vi "Sensors_GCFS.vi"(0 "?":T2={"Core"={"Current VI Reference"=refnum, "Close Panel on Exit?"=FALSE}, "Your Boolean data"=FALSE, "Your string data"="", "Camera Cluster"={"Session"="", "Image"=refnum, "Position Image"=refnum, "PixelVal Image"=refnum, "Position Image Binary"=refnum, "Lable Image"=refnum, "Merged Image"=refnum, "Connection"=FALSE}, "Data In Cluster"={"Images"={"Position Image path"=path "", "Sample folder path"=path "", "Label Image path"=path ""}, "Sample Name"="", "Sample Rate"=0, "Gradient Buffer"=0, "Data Acquisition.Setup.TempGrad"=0.0, "Control.PID gains"={"proportional gain (Kc)"=0.0, "integral time (Ti, min)"=0.0, "derivative time (Td, min)"=0.0}, "Freezing value"=250.0}, "Active"=FALSE, "Ready"=FALSE, "Exit"=FALSE, "Arduino"={"Connection"=FALSE, "Port"="", "State"=""}, "Program_Start"="", "Data Out Cluster"={"Particle Measurements"=[], "Number of droplets"=0, "PosImg_Timestamp"="", "OverlayProp"=[], "Group"="", "Que"=refnum}, "PSU"={"Connection"=FALSE, "Port"="", "State"=""}, "Load Rerun"=FALSE, "Rerun"=FALSE, "cDAQ"={"Connection"=FALSE, "ID"="", "Task"=""}} {"Data Out Cluster"."Particle Measurements" format="%.2f"}, 7 "CheckResponse?":bool, 9 "reinitialize? (F)":bool, 11 "error in":errorcluster) -> (1 "Image Out":T1, 2 "date/time string":string, 3 "Temperature":dbl, 6 "Freezing data":bool, 8 "Freezing_points":string[](array[string]), 10 "Value_Array":string[](array[string]), 14 "valid?":bool, 15 "error out":errorcluster)   [LabVIEW 2024]
uses:
  Micro/DataCluster_GCFS.ctl
  <vilib>/userDefined/High Color/IMAQdx.ctl
  <vilib>/vision/Image Controls.llb/IMAQ Image.ctl
  <vilib>/vision/Image Controls.llb/Overlay Property.ctl
panel:
  in  "Manual Temp Control.Active":bool
  out "Output%":dbl format="%.2f"
  out "Temp Gradient":dbl
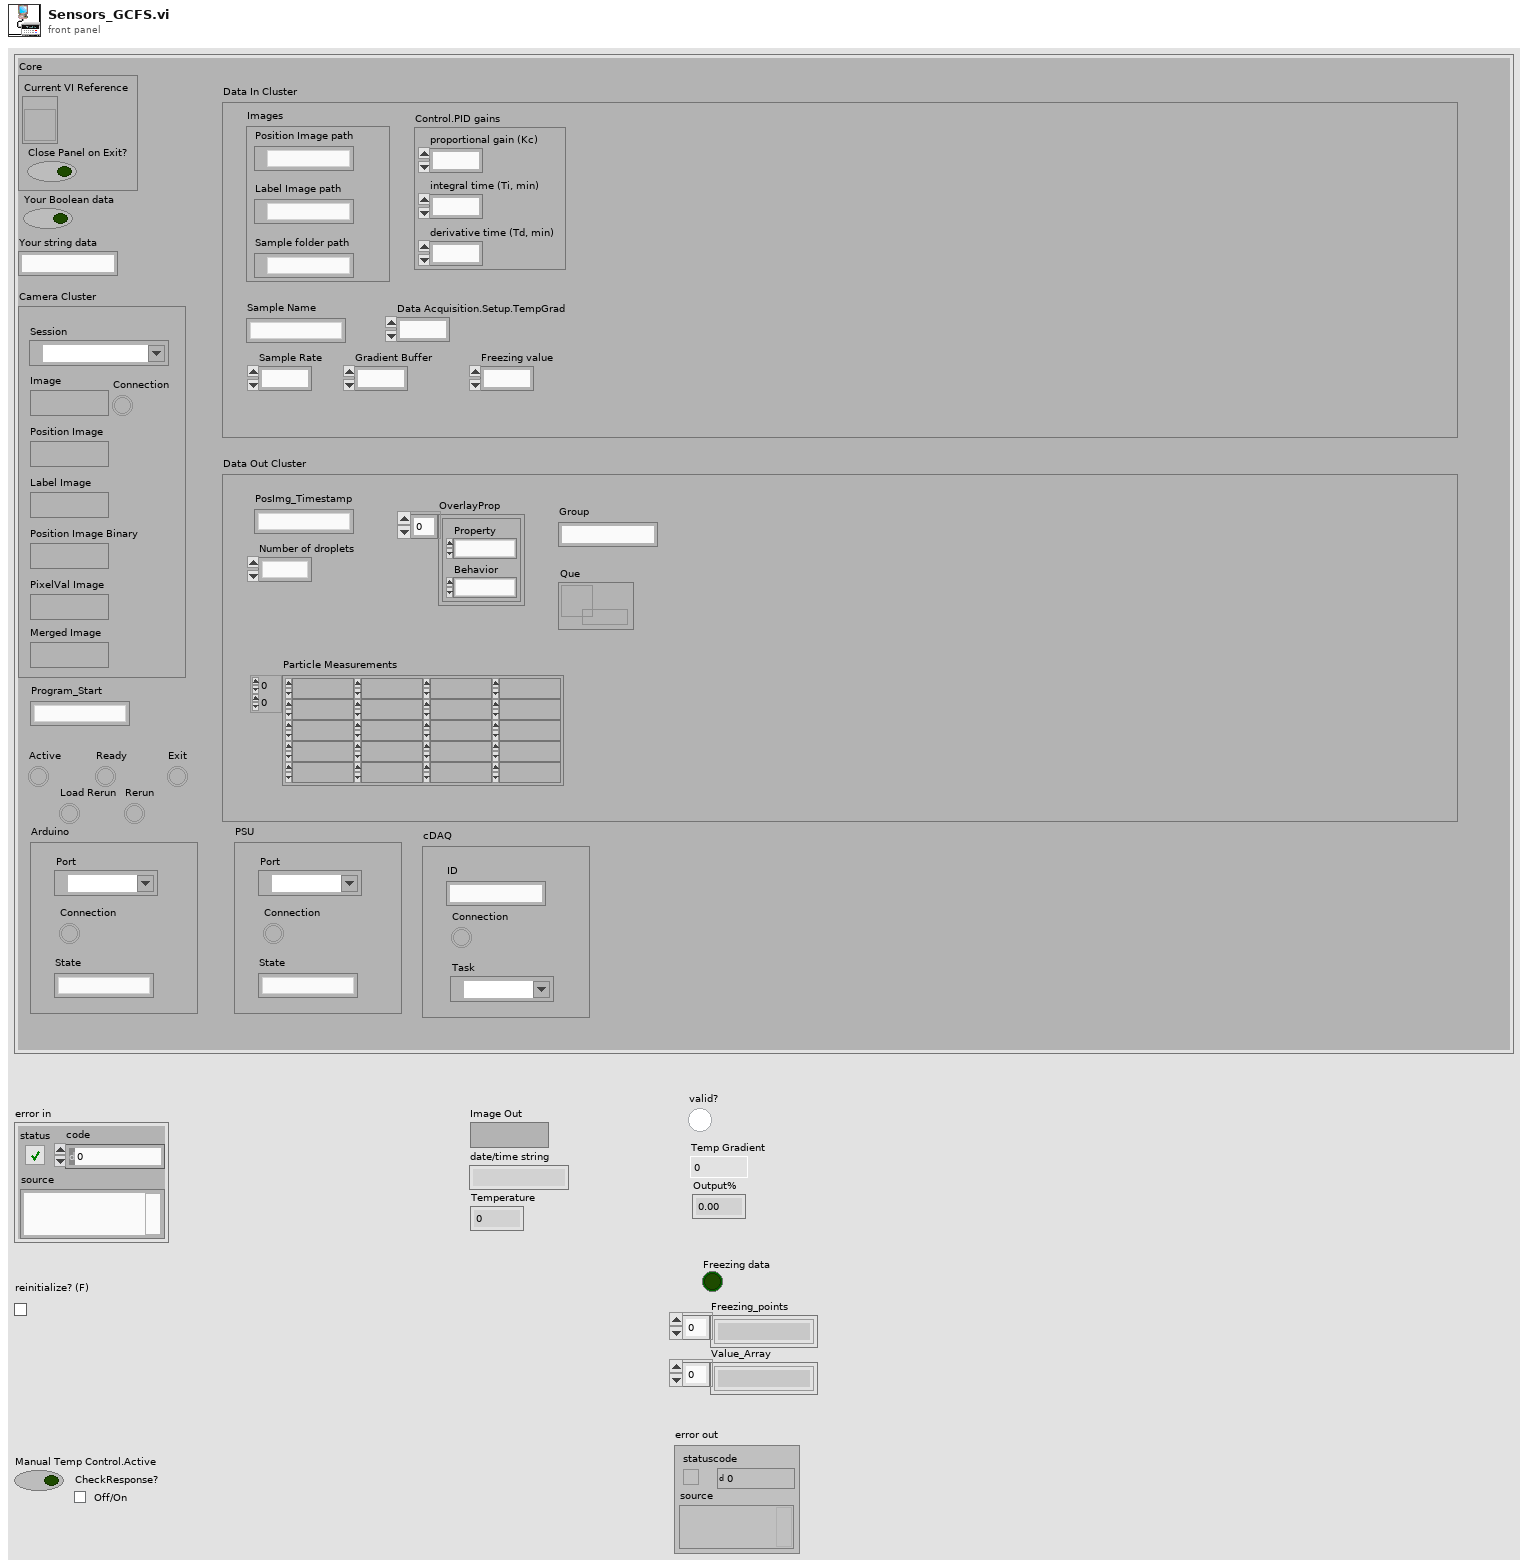
[diagram p1: front panel]
types:
  T1 = typedef "IMAQ Image.ctl" = refnum<image>
  T2 = typedef "DataCluster_GCFS.ctl" = cluster{"Core":cluster{"Current VI Reference":refnum<vi>, "Close Panel on Exit?":bool}, "Your Boolean data":bool, "Your string data":string, "Camera Cluster":cluster{"Session":T3, "Image":T1, "Position Image":T1, "PixelVal Image":T1, "Position Image Binary":T1, "Lable Image":T1, "Merged Image":T1, "Connection":bool}, "Data In Cluster":cluster{"Images":cluster{"Position Image path":path, "Sample folder path":path, "Label Image path":path}, "Sample Name":string, "Sample Rate":i32, "Gradient Buffer":i32, "Data Acquisition.Setup.TempGrad":dbl, "Control.PID gains":cluster{"proportional gain (Kc)":dbl, "integral time (Ti, min)":dbl, "derivative time (Td, min)":dbl}, "Freezing value":sgl}, "Active":bool, "Ready":bool, "Exit":bool, "Arduino":cluster{"Connection":bool, "Port":refnum<visa-resource-name>, "State":string}, "Program_Start":string, "Data Out Cluster":cluster{"Particle Measurements":dbl[][], "Number of droplets":i32, "PosImg_Timestamp":string, "OverlayProp":T4[], "Group":string, "Que":refnum<queue>}, "PSU":cluster{"Connection":bool, "Port":refnum<visa-resource-name>, "State":string}, "Load Rerun":bool, "Rerun":bool, "cDAQ":cluster{"Connection":bool, "ID":string, "Task":refnum<k21>}}
  T3 = typedef "IMAQdx.ctl" = refnum<k21>
  T4 = typedef "Overlay Property.ctl" = cluster{"Property":enum32{"Scale", "Shift", "Rotate", "Symmetry"}, "Behavior":enum32{"Clear", "Keep", "Transform"}}
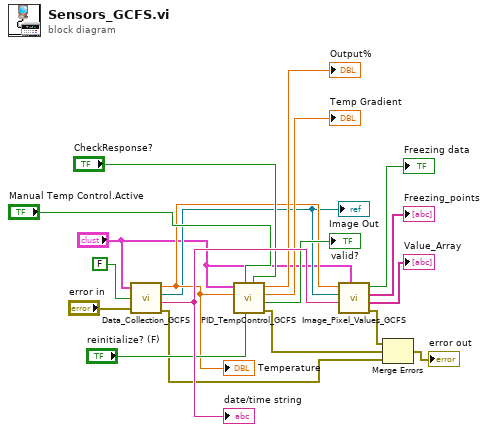
[diagram p0: block diagram]
diagram:
  n1 = call "Data_Collection_GCFS.vi"(0:"?", "Droplet num"=FALSE, "error in"="error in") -> ("Temperature"=w7:dbl, "Image Out"=w6:T1, "date/time string"=w15:string, "error out"=w2:errorcluster)
  "Image Out" <- w6
  "Temperature" <- w7
  "date/time string" <- w15
  n2 = call "PID_TempControl_GCFS.vi"("CheckResponse?"="CheckResponse?", "reinitialize? (F)"="reinitialize? (F)", "Manual Temp Control.Active"="Manual Temp Control.Active", "Temperature"=w7, 11:"?") -> ("error out"=w3:errorcluster, "valid?"=→"valid?":bool, "Temp Gradient"=→"Temp Gradient":dbl, "Output%"=→"Output%":dbl)  [unwired: 3 in]
  n3 = call "Image_Pixel_Values_GCFS.vi"(4:"?", "date/time string"=w15, "Image in"=w6, "Temperature"=w7) -> ("error out"=w4:errorcluster, "Value_Array"=→"Value_Array":string[], "Freezing_points"=→"Freezing_points":string[], "Freezing data"=→"Freezing data":bool)  [unwired: 1 in]
  n4 = Merge Errors(w4, w3, w2) -> (→"error out":errorcluster)
